vi "ChkFldrByAppDir.vi"(8 "error in (no error)":errorcluster, 10 "Folder Name":string, 11 "Rel. Path":path) -> (0 "error out":errorcluster, 2 "file or folder exists?":bool)   [LabVIEW 2020, in "CameraI2COUSB.lvlib" / "CameraDemo.lvclass"]
uses:
  CameraDemo.lvclass
  CameraDemo.lvclass/CameraDemo.ctl
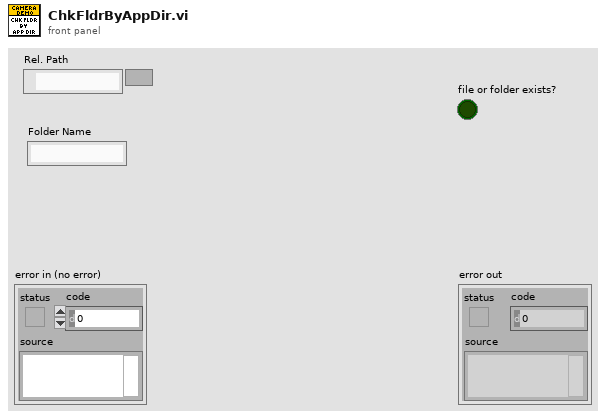
[diagram p1: front panel]
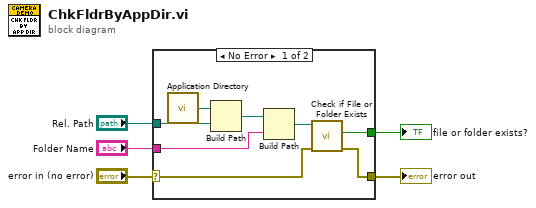
[diagram p0: block diagram]
diagram:
  n1 = case shown="No Error" "error in (no error)" {
    selector: "error in (no error)" -> [w8 w14]
    tunnel: [w7 w14] -> w4
    tunnel: "Rel. Path" -> [w10 _]
    tunnel: "Folder Name" -> [w9 _]
    tunnel: [w6 _] -> w1
    frame No Error {
      n2 = call <vilib>:"Application Directory.vi"() -> ("Application Directory"=w13:path)
      n3 = Build Path(base path=w13, name or relative path=w10) -> (appended path=w12:path)
      n4 = Build Path(base path=w12, name or relative path=w9) -> (appended path=w11:path)
      n5 = call <vilib>:"Check if File or Folder Exists.vi"("error in (no error)"=w8, "path"=w11) -> ("error out"=w7:errorcluster, "file or folder exists?"=w6:bool)  [unwired: 7 in, 1 out]
    }
    frame Error {
    }
  }
  "error out" <- w4
  "file or folder exists?" <- w1
